vi "Revision Query.vi"(8 "error in (no error)":errorcluster, 11 "VISA resource name":refnum<visa-resource-name>) -> (0 "error out":errorcluster, 1 "Instrument Firmware Revision":string, 2 "Instrument Driver Revision":string, 3 "VISA resource name out":refnum<visa-resource-name>)   [LabVIEW 2020, in "Andeen-Hagerling 2700A.lvlib"]
doc: "Queries the current instrument firmware revision and instrument driver revision."
uses:
  Andeen-Hagerling 2700A.lvlib
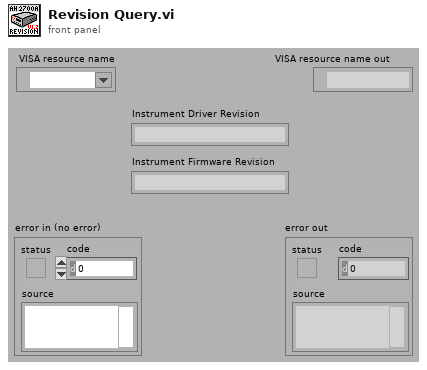
[diagram p1: front panel]
types:
  T1 = cluster{"Major":u16, "Minor":u16, "Fix":u16, "Build":u16}
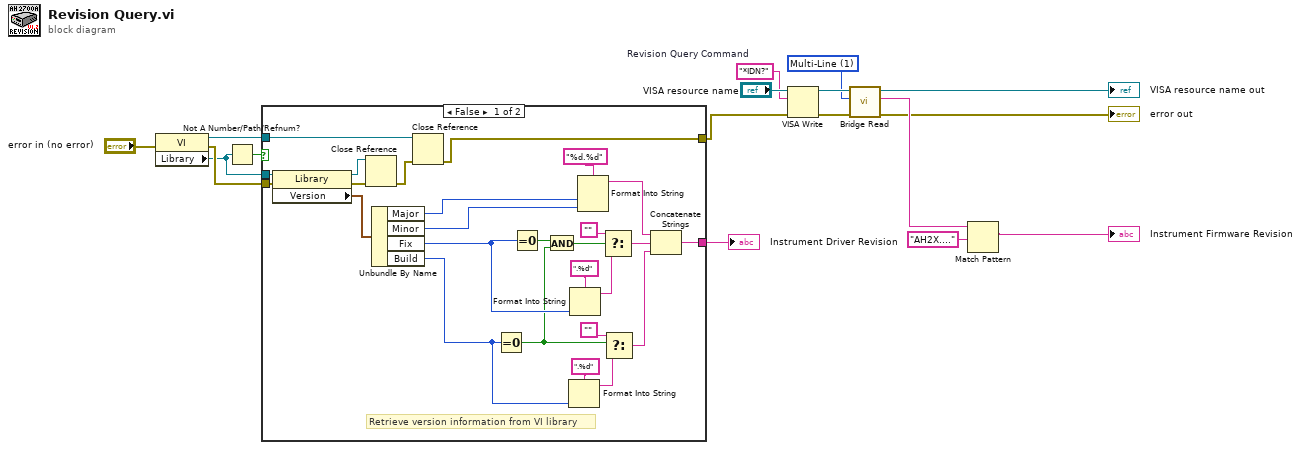
[diagram p0: block diagram]
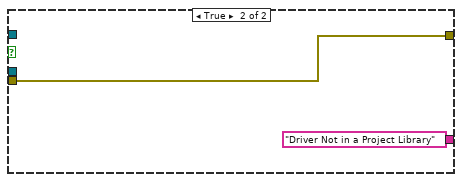
[diagram p2: hidden frame]
diagram:
  w3 = u16 1 items=["Single Line", "Multi-Line"] ("Multiline")
  w14 = "*IDN?"  # Revision Query Command
  n1 = property class="VI"(error in="error in (no error)") -> (reference out=w13:refnum<vi>, error out=w12:errorcluster, "Library"=w11:refnum<vi>)  [unwired: 1 in]
  n2 = Not A Number/Path/Refnum?(number/path/refnum=w11) -> (NaN/Path/Refnum?=w10:bool)
  n3 = case shown="False" w10 {
    tunnel: w13 -> [w40 _]
    tunnel: w12 -> [w25 w45]
    tunnel: [w20 w45] -> w7
    tunnel: [w19 "Driver Not in a Project Library"] -> w9
    tunnel: w11 -> [w18 _]
    frame False {
      # "Retrieve version information from VI library"
      n4 = property class="Library"(reference=w18, error in=w25) -> (reference out=w42:refnum<vi>, error out=w43:errorcluster, "Version"=w39:T1)
      n5 = Close Reference(reference=w42, error in (no error)=w43) -> (error out=w41:errorcluster)
      n6 = Unbundle By Name(w39) -> ("Major"=w28:u16, "Minor"=w27:u16, "Fix"=w24:u16, "Build"=w26:u16)
      n7 = Close Reference(reference=w40, error in (no error)=w41) -> (error out=w20:errorcluster)
      n8 = Equal To 0?(x=w26) -> (x = 0?=w22:bool)
      n9 = Equal To 0?(x=w24) -> (x = 0?=w23:bool)
      n10 = And(x=w23, y=w22) -> (x .and. y?=w21:bool)
      n11 = Format Into String(format string=".%d", w26) -> (resulting string=w32:string)  [unwired: 2 in, 1 out]
      n12 = Format Into String(format string=".%d", w24) -> (resulting string=w36:string)  [unwired: 2 in, 1 out]
      n13 = Format Into String(format string="%d.%d", w28, w27) -> (resulting string=w34:string)  [unwired: 2 in, 1 out]
      n14 = Select(t="", s=w21, f=w36) -> (s? t:f=w33:string)
      n15 = Select(t="", s=w22, f=w32) -> (s? t:f=w29:string)
      n16 = Concatenate Strings(w34, w33, w29) -> (w19:string)
    }
    frame True {
    }
  }
  "Instrument Driver Revision" <- w9
  n17 = VISA Write(VISA resource name="VISA resource name", write buffer=w14, error in (no error)=w7) -> (VISA resource name out=w16:refnum<visa-resource-name>, error out=w15:errorcluster)  [unwired: 1 out]
  n18 = call "Bridge Read.vi"("error in (no error)"=w15, "multiline"=w3, "VISA resource name"=w16) -> ("error out"=→"error out":errorcluster, "read buffer"=w4:string, "VISA resource name out"=→"VISA resource name out":refnum<visa-resource-name>)  [unwired: 6 in]
  n19 = Match Pattern(string=w4, regular expression="AH2X....") -> (match substring=→"Instrument Firmware Revision":string)  [unwired: 1 in, 3 out]
